vi "ChapR cRIO Translater.vi"(6 "Position":u8=49, 7 "CMD":u8, 8 "Alliance":u8=66, 10 "ChapR Data":string, 11 "TeamNo":u16) -> (2 "Network Data":string)   [LabVIEW 2013]
uses:
  ChapR Packet.ctl
  Driver Station Packet.ctl
panel:
  in  "Network Packet":T1
  in  "ChapR Packet":T2
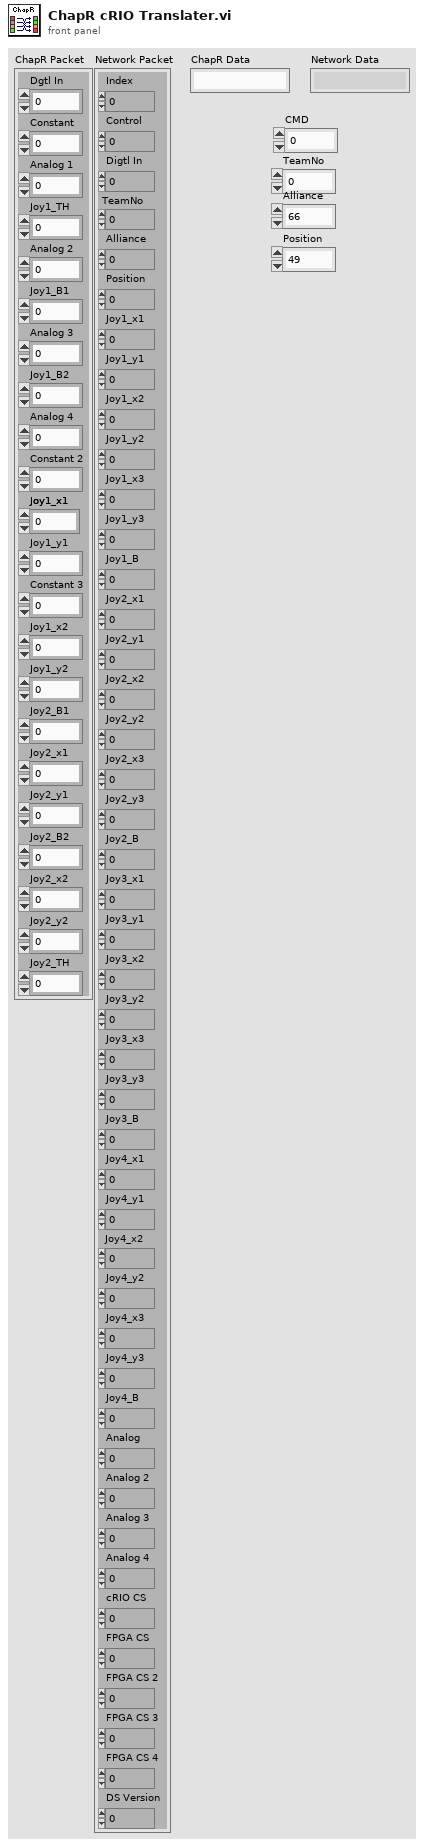
[diagram p1: front panel]
types:
  T1 = typedef "Driver Station Packet.ctl" = cluster{"Index":u16, "Control":u8, "Digtl In":u8, "TeamNo":u16, "Alliance":u8, "Position":u8, "Joy1_x1":i8, "Joy1_y1":i8, "Joy1_x2":i8, "Joy1_y2":i8, "Joy1_x3":i8, "Joy1_y3":i8, "Joy1_B":u16, "Joy2_x1":i8, "Joy2_y1":i8, "Joy2_x2":i8, "Joy2_y2":i8, "Joy2_x3":i8, "Joy2_y3":i8, "Joy2_B":u16, "Joy3_x1":i8, "Joy3_y1":i8, "Joy3_x2":i8, "Joy3_y2":i8, "Joy3_x3":i8, "Joy3_y3":i8, "Joy3_B":u16, "Joy4_x1":i8, "Joy4_y1":i8, "Joy4_x2":i8, "Joy4_y2":i8, "Joy4_x3 ":i8, "Joy4_y3":i8, "Joy4_B":u16, "Analog":u16, "Analog 2":u16, "Analog 3":u16, "Analog 4":u16, "cRIO CS":u64, "FPGA CS":u32, "FPGA CS 2":u32, "FPGA CS 3":u32, "FPGA CS 4":u32, "DS Version":u64}
  T2 = typedef "ChapR Packet.ctl" = cluster{"Dgtl In":u8, "Constant":u8, "Analog 1":u16, "Joy1_TH":u8, "Analog 2":u16, "Joy1_B1":u8, "Analog 3":u16, "Joy1_B2":u8, "Analog 4":u16, "Constant 2":u8, "Joy1_x1":i8, "Joy1_y1":i8, "Constant 3":u8, "Joy1_x2":i8, "Joy1_y2":i8, "Joy2_B1":u8, "Joy2_x1":i8, "Joy2_y1":i8, "Joy2_B2":u8, "Joy2_x2":i8, "Joy2_y2":i8, "Joy2_TH":u8}
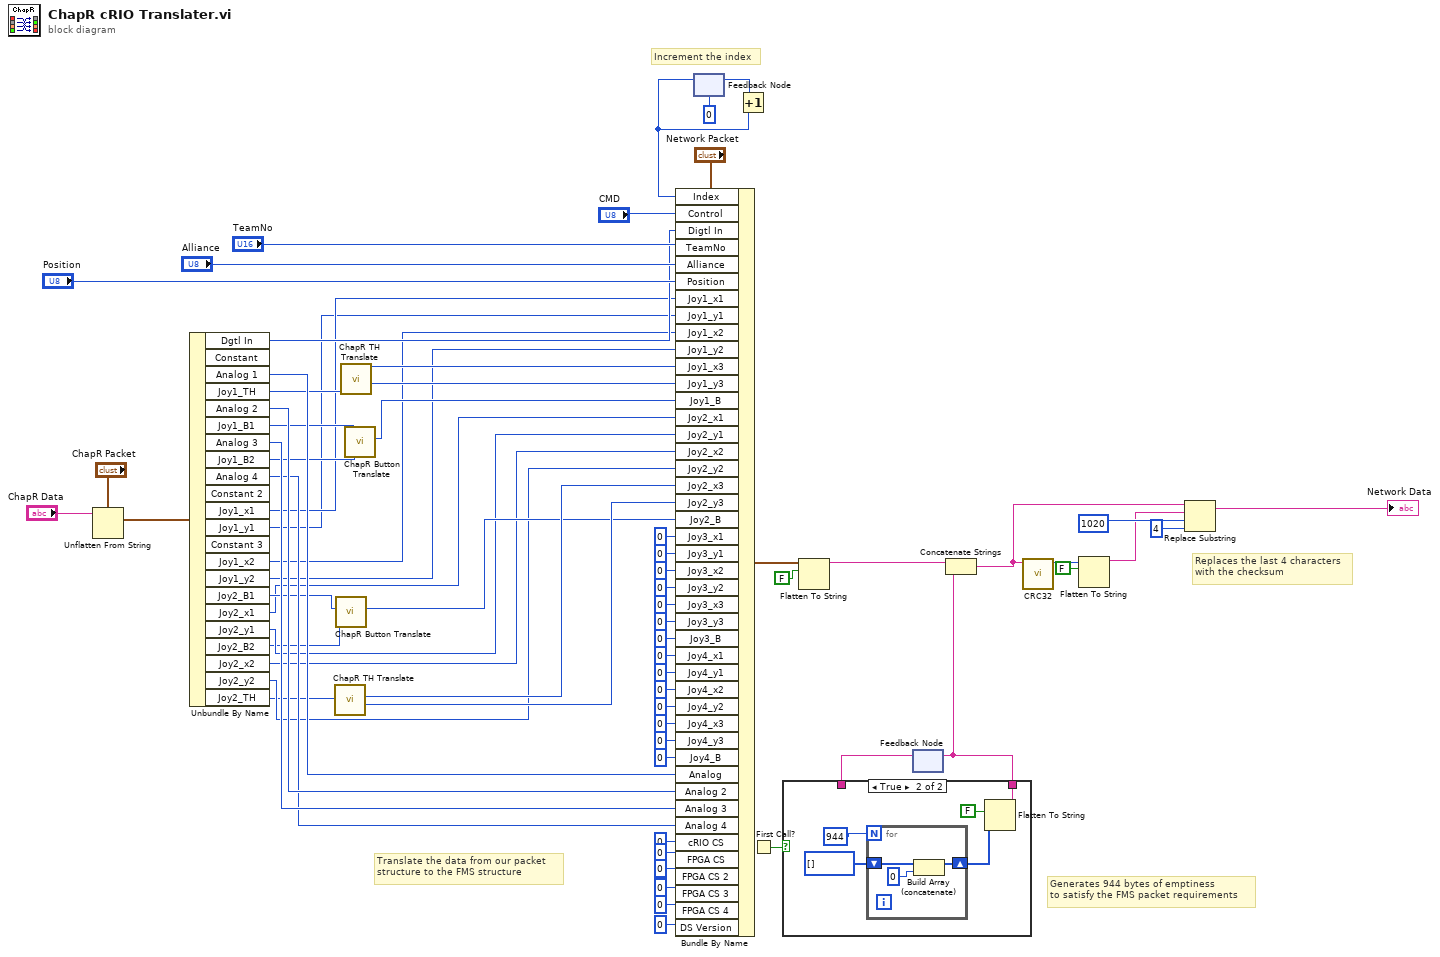
[diagram p0: block diagram]
diagram:
  # "Increment the index"
  # "Translate the data from our packet \nstructure to the FMS structure"
  # "Replaces the last 4 characters \nwith the checksum"
  # "Generates 944 bytes of emptiness \nto satisfy the FMS packet requirements"
  n1 = Unflatten From String(type="ChapR Packet", binary string="ChapR Data") -> (value=w67:T2)  [unwired: 3 in, 2 out]
  n2 = Unbundle By Name(w67) -> ("Dgtl In"=w19:u8, "Analog 1"=w18:u16, "Joy1_TH"=w17:u8, "Analog 2"=w16:u16, "Joy1_B1"=w15:u8, "Analog 3"=w14:u16, "Joy1_B2"=w13:u8, "Analog 4"=w12:u16, "Joy1_x1"=w11:i8, "Joy1_y1"=w10:i8, "Joy1_x2"=w9:i8, "Joy1_y2"=w8:i8, "Joy2_B1"=w7:u8, "Joy2_x1"=w1:i8, "Joy2_y1"=w6:i8, "Joy2_B2"=w5:u8, "Joy2_x2"=w4:i8, "Joy2_y2"=w3:i8, "Joy2_TH"=w2:u8)  [unwired: 3 out]
  n3 = call "ChapR TH Translate.vi"("Tophat Value"=w2) -> ("Y"=w62:i8, "X"=w61:i8)  [unwired: 9 in]
  n4 = call "ChapR Button Translate.vi"("B2"=w5, "B1"=w7) -> ("B"=w39:u16)  [unwired: 9 in]
  n5 = call "ChapR TH Translate.vi"("Tophat Value"=w17) -> ("Y"=w63:i8, "X"=w64:i8)  [unwired: 9 in]
  n6 = call "ChapR Button Translate.vi"("B2"=w13, "B1"=w15) -> ("B"=w60:u16)  [unwired: 9 in]
  n7 = feedback #1(u16 0) -> (w37:u16)
  n8 = Bundle By Name(cluster="Network Packet", "Index"=w37, "Control"="CMD", "Digtl In"=w19, "TeamNo"="TeamNo", "Alliance"="Alliance", "Position"="Position", "Joy1_x1"=w11, "Joy1_y1"=w10, "Joy1_x2"=w9, "Joy1_y2"=w8, "Joy1_x3"=w64, "Joy1_y3"=w63, "Joy1_B"=w60, "Joy2_x1"=w1, "Joy2_y1"=w6, "Joy2_x2"=w4, "Joy2_y2"=w3, "Joy2_x3"=w61, "Joy2_y3"=w62, "Joy2_B"=w39, "Joy3_x1"=i8 0, "Joy3_y1"=i8 0, "Joy3_x2"=i8 0, "Joy3_y2"=i8 0, "Joy3_x3"=i8 0, "Joy3_y3"=i8 0, "Joy3_B"=u16 0, "Joy4_x1"=i8 0, "Joy4_y1"=i8 0, "Joy4_x2"=i8 0, "Joy4_y2"=i8 0, "Joy4_x3"=i8 0, "Joy4_y3"=i8 0, "Joy4_B"=u16 0, "Analog"=w18, "Analog 2"=w16, "Analog 3"=w14, "Analog 4"=w12, "cRIO CS"=u64 0, "FPGA CS"=u32 0, "FPGA CS 2"=u32 0, "FPGA CS 3"=u32 0, "FPGA CS 4"=u32 0, "DS Version"=u64 0) -> (w66:T1)
  n9 = Increment(x=w37) -> (x+1=w36:u16)
  n10 = feedback-in #1(w36) -> ()
  n11 = First Call?() -> (First Call?: T/F=w26:bool)
  n12 = Flatten To String(anything=w66, prepend array or string size? (T)=FALSE) -> (data string=w23:string)  [unwired: 2 in, 2 out]
  n13 = feedback #2() -> (w25:string)  [unwired: 1 in]
  n14 = case shown="True" w26 {
    tunnel: [w70 w72] -> w22
    tunnel: w25 -> [w70 _]
    frame False {
    }
    frame True {
      n15 = for {
        N: 944 -> [_]
        shift-right: [w76] -> w73
        shift-left: u8[] [] -> [w78]
        n16 = Build Array (concatenate)(w78, u8 0) -> (w76:u8[])
      }
      n17 = Flatten To String(anything=w73, prepend array or string size? (T)=FALSE) -> (data string=w72:string)  [unwired: 2 in, 2 out]
    }
  }
  n18 = feedback-in #2(w22) -> ()
  n19 = Concatenate Strings(w23, w22) -> (w24:string)
  n20 = call "CRC32.vi"("Data"=w24) -> ("CRC32Value"=w30:u32)  [unwired: 10 in]
  n21 = Flatten To String(anything=w30, prepend array or string size? (T)=FALSE) -> (data string=w29:string)  [unwired: 2 in, 2 out]
  n22 = Replace Substring(2:4 ("length (len. of substring)"), 3:1020 ("offset (0)"), 4:w29, 5:w24) -> (1:→"Network Data":string)  [unwired: 1 out]
